vi "Send Notification.vi"(8 "error in (no error)":errorcluster, 9 "Code (0)":i32, 10 "Notification Type (Notification)":T2=enum."Notification", 11 "Description (\"\")":string) -> (0 "error out":errorcluster, 3 "Notification":T1)   [LabVIEW 2023]
uses:
  Type Definitions/Enum - Notification Types.ctl
  Type Definitions/Notification Data.ctl
  Type Definitions/Payload Class.ctl
  Type Definitions/Enum - Data.ctl
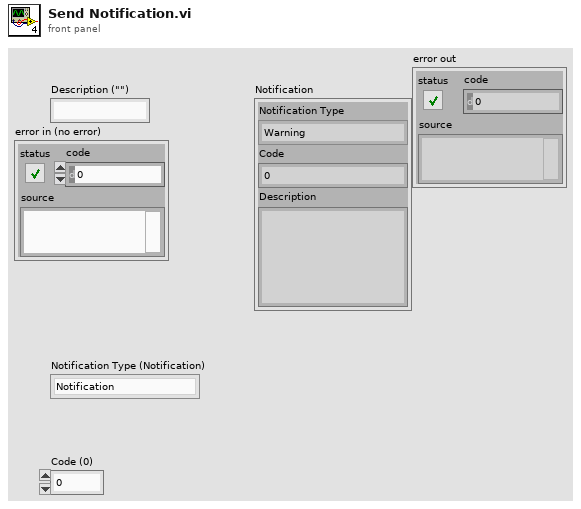
[diagram p1: front panel]
types:
  T1 = typedef "Notification Data.ctl" = cluster{"Notification Type":T2, "Code":i32, "Description":string}
  T2 = typedef "Enum - Notification Types.ctl" = enum16{"Warning", "Acknowledge", "Notification"}
  T3 = typedef "Enum - Data.ctl" = enum16{"Analog Input Data", "Notification Data", "Analog Output Data", "Digital Output Data", "Command Ack", "Digital Input Data", "GPS Solution Data"}
  T4 = typedef "Payload Class.ctl" = enum16{"System State", "Parameters", "Metadata", "Software Monitor", "Data", "Commands"}
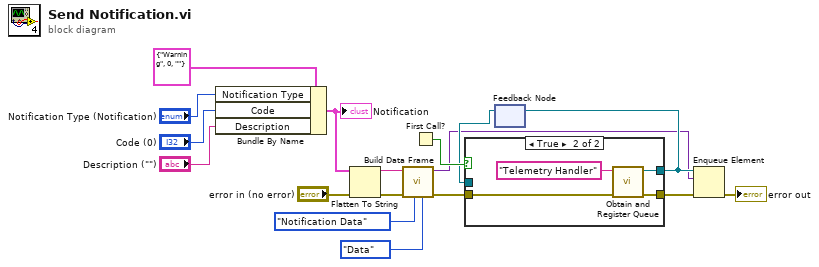
[diagram p0: block diagram]
diagram:
  n1 = Bundle By Name(cluster=T1 {"Notification Type"=enum."Warning", "Code"=0, "Description"=""} ("Notification Data"), "Notification Type"="Notification Type (Notification)", "Code"="Code (0)", "Description"="Description (\"\")") -> (w15:T1)
  "Notification" <- w15
  n2 = Flatten To String(anything=w15, error in (no error)="error in (no error)") -> (data string=w16:string, error out=w17:errorcluster)  [unwired: 2 in, 1 out]
  n3 = call "Build Data Frame.vi"("Payload Class (Data)"=Payload_Class."Data", "Payload ID (0)"=Enum_-_Data."Notification Data" ("Data"), "error in (no error)"=w17, "Payload (Empty String)"=w16) -> ("error out"=w2:errorcluster, "Frame"=w5:variant)  [unwired: 6 in]
  n4 = First Call?() -> (First Call?: T/F=w8:bool)
  n5 = feedback #1() -> (w7:refnum<queue>)  [unwired: 1 in]
  n6 = case shown="True" w8 {
    tunnel: [w19 w22] -> w6
    tunnel: w7 -> [w19 _]
    tunnel: w2 -> [w18 w21]
    tunnel: [w18 w20] -> w1
    frame False {
    }
    frame True {
      n7 = call "Obtain and Register Queue.vi"("error in (no error)"=w21, "Queue Name (unnamed)"="Telemetry Handler" ("name (unnamed)")) -> ("error out"=w20:errorcluster, "Queue Reference"=w22:refnum<queue>)  [unwired: 8 in]
    }
  }
  n8 = feedback-in #1(w6) -> ()
  n9 = Enqueue Element(queue=w6, element=w5, error in (no error)=w1) -> (error out=→"error out":errorcluster)  [unwired: 1 in, 2 out]
